vi "Begin.vi"(8 "error in":errorcluster) -> (0 "error out":errorcluster)   [LabVIEW 2015]
doc: "Called before other user functions, this VI is expected to open initial I/O refnums, load in file data, and do all program initialization. Notice that the <B>error out</B> terminal is simply used for data flow. Wiring it to other structures or subVIs ensures that this VI runs first."
uses:
  <vilib>/Rock Robotics/WPI/DriverStation/WPI_DriverStationRobotMode2.ctl
  <vilib>/Rock Robotics/WPI/Joystick/WPI_JoystickDeviceEnum.ctl
  <vilib>/Rock Robotics/SystemInterfaces/DIO/FPGA_DIOChannel.ctl
  <vilib>/Rock Robotics/WPI/CAN/TalonSRX/WPI_CANTalonSRX_APIControlMode.ctl
  <vilib>/Rock Robotics/SystemInterfaces/DIO/FPGA_DIOPWMChannel.ctl
  <vilib>/Rock Robotics/WPI/CAN/TalonSRX/WPI_CANTalonSRX_BrakeOverride.ctl
  <vilib>/Rock Robotics/WPI/CAN/TalonSRX/WPI_CANTalonSRX_APIFeedbackSelect.ctl
  Robot Global Data.vi
  <vilib>/Rock Robotics/Network Tables/NT Write String Array.vi
  <vilib>/Rock Robotics/WPI/MotorControl/WPI_MotorControlOpenCANTalonSRX.vi
  <vilib>/Rock Robotics/WPI/RobotDrive/WPI_RobotDriveOpen4MotorWithTalon.vi
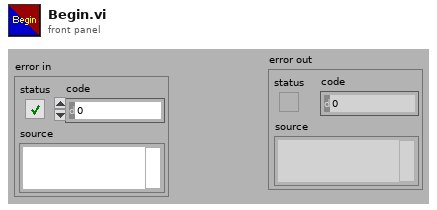
[diagram p1: front panel]
types:
  T1 = typedef "WPI_CANTalonSRX_APIFeedbackSelect.ctl" = enum16{"Digital Quadrature Encoder", "Analog Potentiometer", "Analog Encoder", "Count on Quad-A (Rising-Edge)", "Count on Quad-A (Falling-Edge)", "CTR Magnetic Enc (Absolute)", "CTR Magnetic Enc (Relative)", "Pulse Width"}
  T2 = typedef "WPI_CANTalonSRX_BrakeOverride.ctl" = enum8{"No Override", "Override to Coast", "Override to Brake"}
  T3 = typedef "WPI_CANTalonSRX_APIControlMode.ctl" = enum8{"Percent VBus", "Speed", "Position", "Slave", "Unchanged / Invalid", "Voltage Compensation", "Current", "Motion Profile"}
  T4 = typedef "FPGA_DIOPWMChannel.ctl" = enum8{"PWM 0", "PWM 1", "PWM 2", "PWM 3", "PWM 4", "PWM 5", "PWM 6", "PWM 7", "PWM 8", "PWM 9", "PWM MXP 0", "PWM MXP 1", "PWM MXP 2", "PWM MXP 3", "PWM MXP 4", "PWM MXP 5", "PWM MXP 6", "PWM MXP 7", "PWM MXP 8", "PWM MXP 9", "Invalid"}
  T5 = typedef "FPGA_DIOChannel.ctl" = enum8{"DIO 0", "DIO 1", "DIO 2", "DIO 3", "DIO 4", "DIO 5", "DIO 6", "DIO 7", "DIO 8", "DIO 9", "DIO MXP 0", "DIO MXP 1", "DIO MXP 2", "DIO MXP 3", "DIO MXP 4", "DIO MXP 5", "DIO MXP 6", "DIO MXP 7", "DIO MXP 8", "DIO MXP 9", "DIO MXP 10", "DIO MXP 11", "DIO MXP 12", "DIO MXP 13", "DIO MXP 14", "DIO MXP 15", "Invalid"}
  T6 = typedef "WPI_JoystickDeviceEnum.ctl" = enum16{"USB 0", "USB 1", "USB 2", "USB 3", "USB 4", "USB 5"}
  T7 = typedef "WPI_DriverStationRobotMode2.ctl" = enum16{"Autonomous Disabled", "Autonomous Enabled", "Teleop Disabled", "Teleop Enabled", "Disconnected", "Finish", "Test Disabled", "Test Enabled", "Emergency Stopped"}
  T8 = typedef "WPI_JoystickDevRef.ctl" = cluster{"Device":T6}
  T9 = typedef "WPI_DigitalInputDevRef.ctl" = cluster{"DevStatus":errorcluster, "DIO Channel":T5}
  T10 = typedef "WPI_MotorControlDeviceRef.ctl" = cluster{"DeviceStatus":errorcluster, "Type":T11, "PWM":cluster{"PWM Channel":T4, "DeadBand":T12}, "CAN":cluster{"Device Number":u8, "Control Mode":T13, "Semaphore":T14, "Max Vout":dbl, "TalonSRX Control Mode":T3}, "Invert":bool}
  T11 = typedef "WPI_MotorControlType.ctl" = enum16{"PWM", "CAN", "CANTalonSRX"}
  T12 = typedef "WPI_PWMDeadband.ctl" = cluster{"Name":string, "maxPositivePwm":i32, "minPositivePwm":i32, "centerPwm":i32, "maxNegativePwm":i32, "minNegativePwm":i32, "angularRange":u16}
  T13 = typedef "WPI_CANJaguar_ControlMode.ctl" = enum8{"Percent VBus", "Current", "Speed", "Position", "Voltage"}
  T14 = typedef "Semaphore RefNum" = refnum<k1>
  T15 = typedef "WPI_RobotDriveDevRef.ctl" = cluster{"DevStatus":errorcluster, "Motors[]":T10[], "Square Inputs":bool, "Max Output":dbl}
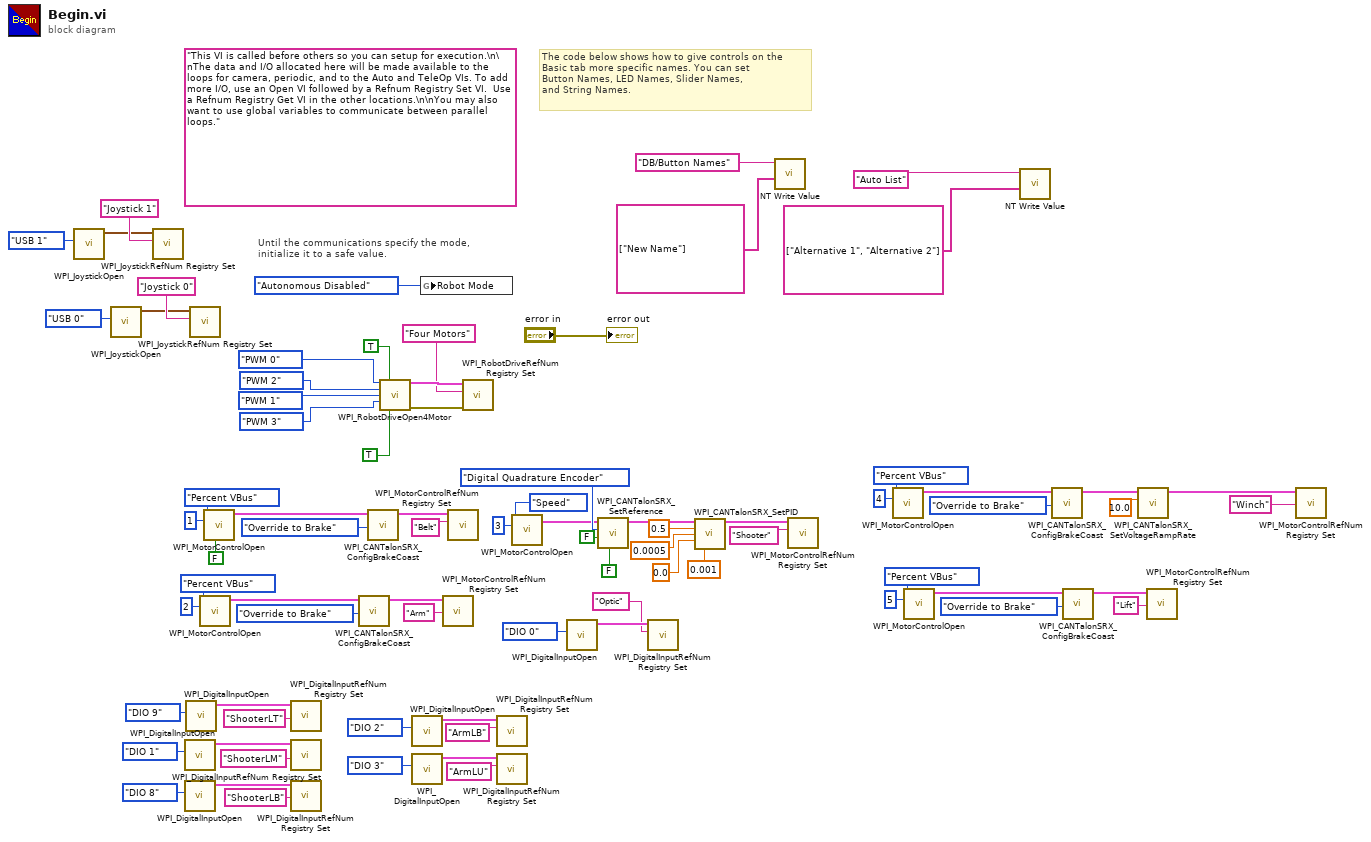
[diagram p0: block diagram]
diagram:
  (unwired) "This VI is called before others so you can setup for execution.\n\nThe data and I/O allocated here will be made available to the loops for camera, periodic, and to the Auto and TeleOp VIs. To add more I/O, use an Open VI followed by a Refnum Registry Set VI.  Use a Refnum Registry Get VI in the other locations.\n\nYou may also want to use global variables to communicate between parallel loops."
  # "The code below shows how to give controls on the\nBasic tab more specific names. You can set\nButton Names, LED Names, Slider Names,\nand String Names."
  # "Until the communications specify the mode,\ninitialize it to a safe value."
  n1 = call <vilib>:"WPI_JoystickOpen.vi"("JoystickDevice"=WPI_JoystickDeviceEnum."USB 1") -> ("JoystickDevRef"=w36:T8)  [unwired: 10 in]
  n2 = call <vilib>:"WPI_JoystickOpen.vi"("JoystickDevice"=WPI_JoystickDeviceEnum."USB 0") -> ("JoystickDevRef"=w74:T8)  [unwired: 10 in]
  n3 = call <vilib>:"WPI_JoystickRefNum Registry Set.vi"("refnum name"="Joystick 1", "JoystickDevRef"=w36) -> ()  [unwired: 8 in, 2 out]
  n4 = call <vilib>:"WPI_DigitalInputOpen.vi"("DIO Channel"=FPGA_DIOChannel."DIO 1") -> ("DigitalInputDevRef"=w65:T9)  [unwired: 9 in, 1 out]
  n5 = call <vilib>:"WPI_DigitalInputOpen.vi"("DIO Channel"=FPGA_DIOChannel."DIO 8") -> ("DigitalInputDevRef"=w67:T9)  [unwired: 9 in, 1 out]
  n6 = call <vilib>:"WPI_DigitalInputOpen.vi"("DIO Channel"=FPGA_DIOChannel."DIO 9") -> ("DigitalInputDevRef"=w62:T9)  [unwired: 9 in, 1 out]
  n7 = call <vilib>:"WPI_JoystickRefNum Registry Set.vi"("refnum name"="Joystick 0", "JoystickDevRef"=w74) -> ()  [unwired: 8 in, 2 out]
  n8 = call-poly <vilib>:"WPI_MotorControlOpen.vi"("Device Number"=u8 2, "Control Mode"=WPI_CANTalonSRX_APIControlMode."Percent VBus") -> ("MotorControlDeviceRef"=w39:T10)  [unwired: 8 in, 1 out]
  n9 = call-poly <vilib>:"WPI_MotorControlOpen.vi"("Invert"=FALSE, "Device Number"=u8 1, "Control Mode"=WPI_CANTalonSRX_APIControlMode."Percent VBus") -> ("MotorControlDeviceRef"=w42:T10)  [unwired: 7 in, 1 out]
  n10 = call <vilib>:"WPI_DigitalInputRefNum Registry Set.vi"("refnum name"="ShooterLT", "DigitalInputDevRef"=w62) -> ()  [unwired: 8 in, 2 out]
  n11 = call <vilib>:"WPI_DigitalInputRefNum Registry Set.vi"("refnum name"="ShooterLM", "DigitalInputDevRef"=w65) -> ()  [unwired: 8 in, 2 out]
  n12 = call <vilib>:"WPI_DigitalInputRefNum Registry Set.vi"("refnum name"="ShooterLB", "DigitalInputDevRef"=w67) -> ()  [unwired: 8 in, 2 out]
  n13 = call <vilib>:"WPI_CANTalonSRX_ConfigBrakeCoast.vi"("Brake / Coast Mode"=WPI_CANTalonSRX_BrakeOverride."Override to Brake", "CAN Talon SRX Ref"=w39) -> ("CAN Talon SRX Ref"=w38:T10)  [unwired: 8 in, 1 out]
  n14 = call <vilib>:"WPI_CANTalonSRX_ConfigBrakeCoast.vi"("Brake / Coast Mode"=WPI_CANTalonSRX_BrakeOverride."Override to Brake", "CAN Talon SRX Ref"=w42) -> ("CAN Talon SRX Ref"=w41:T10)  [unwired: 8 in, 1 out]
  n15 = call-poly <vilib>:"WPI_RobotDriveOpen4Motor.vi"("Rear Left Motor"=FPGA_DIOPWMChannel."PWM 0" ("Left Motor"), "Rear Left Motor Inverted"=TRUE, "Rear Right Motor"=FPGA_DIOPWMChannel."PWM 2" ("Left Motor"), "Front Left Motor"=FPGA_DIOPWMChannel."PWM 1" ("Left Motor"), "Front Right Motor"=FPGA_DIOPWMChannel."PWM 3" ("Left Motor"), "Front Left Motor Inverted"=TRUE) -> ("RobotDriveDevRef"=w79:T15, "error out"=w77:errorcluster)  [unwired: 8 in]
  n16 = call <vilib>:"WPI_DigitalInputOpen.vi"("DIO Channel"=FPGA_DIOChannel."DIO 2") -> ("DigitalInputDevRef"=w54:T9)  [unwired: 9 in, 1 out]
  n17 = call <vilib>:"WPI_DigitalInputOpen.vi"("DIO Channel"=FPGA_DIOChannel."DIO 3") -> ("DigitalInputDevRef"=w51:T9)  [unwired: 9 in, 1 out]
  n18 = global write "Robot Global Data.vi" "Robot Mode"(WPI_DriverStationRobotMode2."Autonomous Disabled" ("Robot Mode")) -> ()
  n19 = call <vilib>:"WPI_MotorControlRefNum Registry Set.vi"("refnum name"="Arm", "MotorControlDevRef"=w38) -> ()  [unwired: 8 in, 2 out]
  n20 = call <vilib>:"WPI_MotorControlRefNum Registry Set.vi"("refnum name"="Belt", "MotorControlDevRef"=w41) -> ()  [unwired: 8 in, 2 out]
  n21 = call <vilib>:"WPI_RobotDriveRefNum Registry Set.vi"("error in (no error)"=w77, "refnum name"="Four Motors", "RobotDriveDevRef"=w79) -> ()  [unwired: 1 in, 8 out]
  n22 = call <vilib>:"WPI_DigitalInputRefNum Registry Set.vi"("refnum name"="ArmLB", "DigitalInputDevRef"=w54) -> ()  [unwired: 8 in, 2 out]
  n23 = call <vilib>:"WPI_DigitalInputRefNum Registry Set.vi"("refnum name"="ArmLU", "DigitalInputDevRef"=w51) -> ()  [unwired: 8 in, 2 out]
  n24 = call-poly <vilib>:"WPI_MotorControlOpen.vi"("Device Number"=u8 3, "Control Mode"=WPI_CANTalonSRX_APIControlMode."Speed") -> ("MotorControlDeviceRef"=w10:T10)  [unwired: 8 in, 1 out]
  n25 = call <vilib>:"WPI_DigitalInputOpen.vi"("DIO Channel"=FPGA_DIOChannel."DIO 0") -> ("DigitalInputDevRef"=w34:T9)  [unwired: 9 in, 1 out]
  n26 = call <vilib>:"WPI_CANTalonSRX_SetReference.vi"("Reverse Closed-Loop Output"=FALSE ("Reverse Feedback Sensor"), "Reverse Feedback Sensor"=FALSE, "Feedback Reference"=WPI_CANTalonSRX_APIFeedbackSelect."Digital Quadrature Encoder", "CAN Talon SRX Ref"=w10) -> ("CAN Talon SRX Ref"=w9:T10)  [unwired: 6 in, 1 out]
  n27 = call <vilib>:"WPI_DigitalInputRefNum Registry Set.vi"("refnum name"="Optic", "DigitalInputDevRef"=w34) -> ()  [unwired: 8 in, 2 out]
  n28 = call <vilib>:"WPI_CANTalonSRX_SetPID.vi"("CAN Talon SRX Ref"=w9, "P"=0.5, "I"=0.0005, "D"=0.0, "F"=0.001) -> ("CAN Talon SRX Ref"=w4:T10)  [unwired: 9 in, 1 out]
  n29 = call-poly <vilib>:"NT Write Value.vi"("String Array"=string[] ["New Name"], "Name"="DB/Button Names") -> ()  [unwired: 9 in, 1 out]
  n30 = call <vilib>:"WPI_MotorControlRefNum Registry Set.vi"("refnum name"="Shooter", "MotorControlDevRef"=w4) -> ()  [unwired: 8 in, 2 out]
  n31 = call-poly <vilib>:"WPI_MotorControlOpen.vi"("Device Number"=u8 4, "Control Mode"=WPI_CANTalonSRX_APIControlMode."Percent VBus") -> ("MotorControlDeviceRef"=w21:T10)  [unwired: 8 in, 1 out]
  n32 = call-poly <vilib>:"WPI_MotorControlOpen.vi"("Device Number"=u8 5, "Control Mode"=WPI_CANTalonSRX_APIControlMode."Percent VBus") -> ("MotorControlDeviceRef"=w16:T10)  [unwired: 8 in, 1 out]
  n33 = call-poly <vilib>:"NT Write Value.vi"("String Array"=string[] ["Alternative 1", "Alternative 2"], "Name"="Auto List") -> ()  [unwired: 9 in, 1 out]
  n34 = call <vilib>:"WPI_CANTalonSRX_ConfigBrakeCoast.vi"("Brake / Coast Mode"=WPI_CANTalonSRX_BrakeOverride."Override to Brake", "CAN Talon SRX Ref"=w21) -> ("CAN Talon SRX Ref"=w14:T10)  [unwired: 8 in, 1 out]
  n35 = call <vilib>:"WPI_CANTalonSRX_ConfigBrakeCoast.vi"("Brake / Coast Mode"=WPI_CANTalonSRX_BrakeOverride."Override to Brake", "CAN Talon SRX Ref"=w16) -> ("CAN Talon SRX Ref"=w15:T10)  [unwired: 8 in, 1 out]
  n36 = call <vilib>:"WPI_CANTalonSRX_SetVoltageRampRate.vi"("Throttle Ramp Rate (percent/s)"=10.0, "CAN Talon SRX Ref"=w14) -> ("CAN Talon SRX Ref"=w12:T10)  [unwired: 8 in, 1 out]
  n37 = call <vilib>:"WPI_MotorControlRefNum Registry Set.vi"("refnum name"="Lift", "MotorControlDevRef"=w15) -> ()  [unwired: 8 in, 2 out]
  n38 = call <vilib>:"WPI_MotorControlRefNum Registry Set.vi"("refnum name"="Winch", "MotorControlDevRef"=w12) -> ()  [unwired: 8 in, 2 out]
  "error out" <- "error in"
